vi "ShowFP.vi"(8 "error in (no error)":errorcluster, 10 "ResetFP":bool caption="Reset Front Panel", 11 "CameraTestingUI in":refnum<class "CameraTestingENI.lvclass">) -> (0 "error out":errorcluster, 3 "CameraTestingUI out":refnum<class "CameraTestingENI.lvclass">)   [LabVIEW 2020, in "CameraTestingProxy.lvlib" / "CameraTestingENI.lvclass"]
uses:
  CameraTestingENI.lvclass
  CameraTestingENI.lvclass/CameraTestingENI.ctl
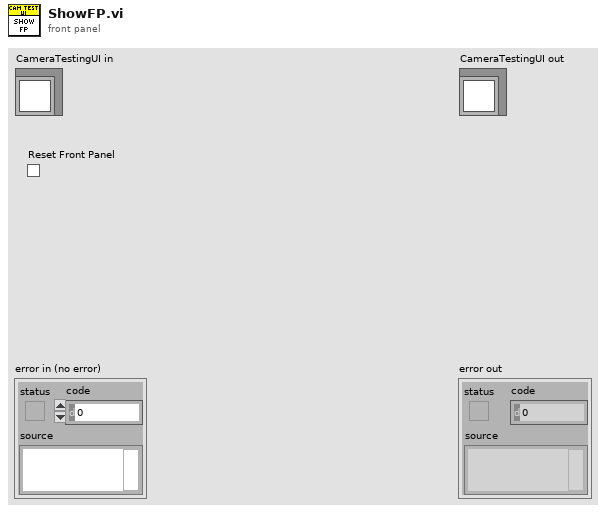
[diagram p1: front panel]
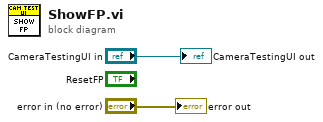
[diagram p0: block diagram]
diagram:
  "error out" <- "error in (no error)"
  "CameraTestingUI out" <- "CameraTestingUI in"
